vi "RunOperation.vi"(10 "Inputs":string[](array[string]), 11 "BuildSolution in":refnum<class "BuildSolution.lvclass">) -> (1 "Output/Failure":string, 2 "CLI Process Return Code":i32, 3 "BuildSolution out":refnum<class "BuildSolution.lvclass">)   [LabVIEW 2019, in "BuildSolution.lvclass"]
uses:
  BuildSolution.lvclass
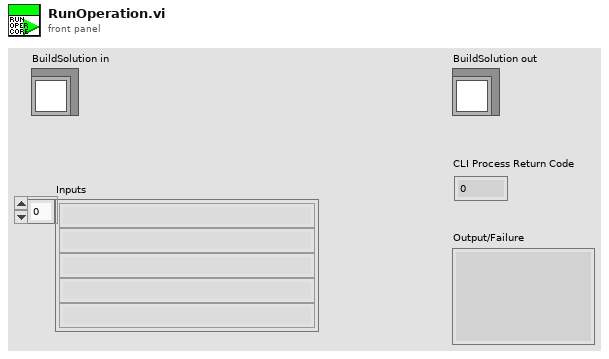
[diagram p1: front panel]
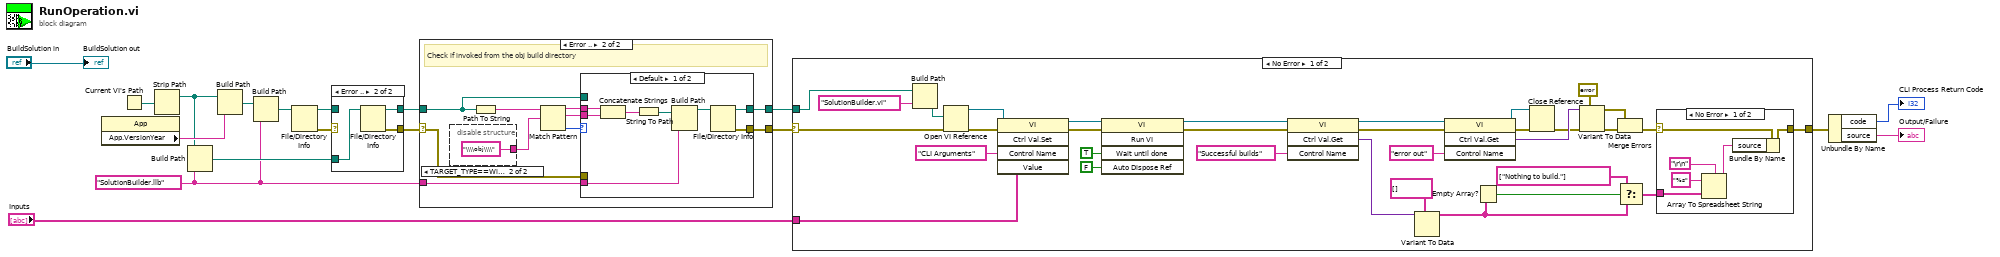
[diagram p0: block diagram]
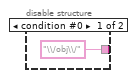
[diagram p5: hidden frame]
diagram:
  w1 = "SolutionBuilder.llb" ("Control Name")
  n1 = property class="App"() -> ("App.VersionYear"=w14:string)  [unwired: 2 in, 2 out]
  n2 = Current VI's Path() -> (path=w15:path)
  n3 = Strip Path(path=w15) -> (stripped path=w12:path)  [unwired: 1 out]
  n4 = Build Path(base path=w12, name or relative path=w1) -> (appended path=w8:path)
  n5 = Build Path(base path=w12, name or relative path=w14) -> (appended path=w13:path)
  n6 = Build Path(base path=w13, name or relative path=w1) -> (appended path=w11:path)
  n7 = File/Directory Info(path=w11) -> (path out=w9:path, error out=w10:errorcluster)  [unwired: 1 in, 5 out]
  n8 = case shown="Error .." w10 {
    selector: w10 -> [w19 _]
    tunnel: w9 -> [w20 _]
    tunnel: [w20 w22] -> w4
    tunnel: [w19 w21] -> w5
    tunnel: w8 -> [_ w23]
    frame No Error {
    }
    frame Error {
      n9 = File/Directory Info(path=w23) -> (path out=w22:path, error out=w21:errorcluster)  [unwired: 1 in, 5 out]
    }
  }
  n10 = case shown="Error .." w5 {
    selector: w5 -> [w24 w26]
    tunnel: w4 -> [w25 w27]
    tunnel: [w25 w35] -> w2
    tunnel: [w24 w34] -> w3
    tunnel: w1 -> [_ w28]
    frame No Error {
    }
    frame Error {
      # "Check if invoked from the obj build directory"
      n11 = disable-structure shown="TARGET_TYPE==Windows" {
        disable-tunnel: ["\\/obj\\/" ("result string") "\\\\obj\\\\" ("result string")] -> w32
        frame condition #0 {
        }
        frame condition #1 (active) {
        }
      }
      n12 = Path To String(path=w27) -> (string=w33:string)
      n13 = Match Pattern(string=w33, regular expression=w32) -> (before substring=w30:string, match substring=w29:string, offset past match=w31:i32)  [unwired: 1 in, 1 out]
      n14 = case shown="Default" w31 {
        tunnel: [w43 w45] -> w35
        tunnel: [w42 w44] -> w34
        tunnel: w30 -> [w41 _]
        tunnel: w29 -> [w40 _]
        tunnel: w28 -> [w36 _]
        tunnel: w27 -> [_ w45]
        tunnel: w26 -> [_ w44]
        frame Default {
          n15 = Concatenate Strings(w41, w40) -> (w39:string)
          n16 = String To Path(string=w39) -> (path=w38:path)
          n17 = Build Path(base path=w38, name or relative path=w36) -> (appended path=w37:path)
          n18 = File/Directory Info(path=w37) -> (path out=w43:path, error out=w42:errorcluster)  [unwired: 1 in, 5 out]
        }
        frame -1 {
        }
      }
    }
  }
  n19 = case shown="No Error" w3 {
    selector: w3 -> [w80 w88]
    tunnel: w2 -> [w62 _]
    tunnel: "Inputs" -> [w77 _]
    tunnel: [w53 w88] -> w6
    frame No Error {
      n20 = Build Path(base path=w62, name or relative path="SolutionBuilder.vi" ("Control Name")) -> (appended path=w63:path)
      n21 = Open VI Reference(vi path=w63, error in (no error)=w80) -> (vi reference=w78:refnum<vi>, error out=w79:errorcluster)  [unwired: 4 in]
      n22 = invoke class="VI" method="Ctrl Val.Set"(reference=w78, error in=w79, "Control Name"="CLI Arguments", "Value"=w77) -> (reference out=w76:refnum<vi>, error out=w75:errorcluster)  [unwired: 1 in, 3 out]
      n23 = invoke class="VI" method="Run VI"(reference=w76, error in=w75, "Wait until done"=TRUE ("Wait Until Done"), "Auto Dispose Ref"=FALSE ("Auto Dispose Reference")) -> (reference out=w59:refnum<vi>, error out=w58:errorcluster)  [unwired: 1 in, 3 out]
      n24 = invoke class="VI" method="Ctrl Val.Get"(reference=w59, error in=w58, "Control Name"="Successful builds") -> (reference out=w57:refnum<vi>, error out=w48:errorcluster, "Get Control Value Variant"=w56:variant)  [unwired: 1 in, 1 out]
      n25 = Variant To Data(type=string[] [] ("Inputs"), Variant=w56) -> (data=w51:string[])  [unwired: 1 in, 1 out]
      n26 = invoke class="VI" method="Ctrl Val.Get"(reference=w57, error in=w48, "Control Name"="error out") -> (reference out=w69:refnum<vi>, error out=w70:errorcluster, "Get Control Value Variant"=w68:variant)  [unwired: 1 in, 1 out]
      n27 = Empty Array?(array=w51) -> (empty?=w52:bool)
      n28 = Close Reference(reference=w69, error in (no error)=w70) -> (error out=w66:errorcluster)
      n29 = Variant To Data(error in=w66, type=errorcluster {"status"=FALSE, "code"=0, "source"=""} ("input cluster"), Variant=w68) -> (data=w64:errorcluster, error out=w65:errorcluster)
      n30 = Merge Errors(w64, w65) -> (w54:errorcluster)
      n31 = Select(t=string[] ["Nothing to build."] ("Inputs"), s=w52, f=w51) -> (s? t:f=w50:string[])
      n32 = case shown="No Error" w54 {
        selector: w54 -> [w86 w87]
        tunnel: [w85 w87] -> w53
        tunnel: w50 -> [w84 _]
        frame No Error {
          n33 = Array To Spreadsheet String(delimiter (Tab)="\r\n", array=w84, 3:"%s" ("format string")) -> (spreadsheet string=w81:string)
          n34 = Bundle By Name(cluster=w86, "source"=w81) -> (w85:errorcluster)
        }
        frame Error {
        }
      }
    }
    frame Error {
    }
  }
  n35 = Unbundle By Name(w6) -> ("code"=→"CLI Process Return Code":i32, "source"=→"Output/Failure":string)
  "BuildSolution out" <- "BuildSolution in"
